vi "2DPlotter.vi"(5 "Reset":bool, 7 "Add":bool, 9 "New Data":i32[][](array[numeric]), 11 "Plot In":i32[][](array[numeric])) -> (3 "Plot Out":i32[][](array[numeric]))   [LabVIEW 2017]
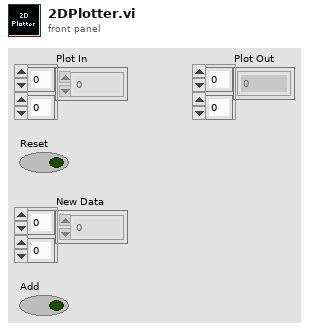
[diagram p1: front panel]
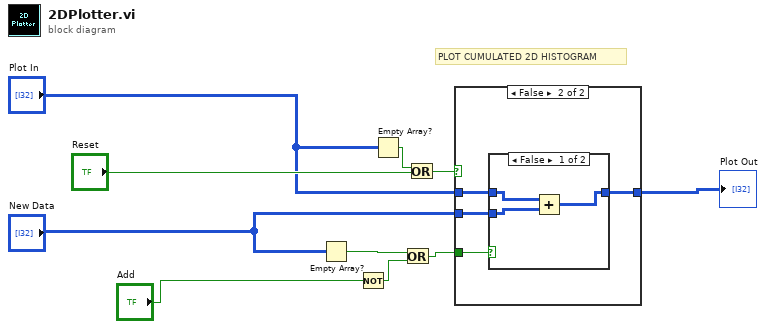
[diagram p0: block diagram]
diagram:
  # "PLOT CUMULATED 2D HISTOGRAM"
  n1 = Empty Array?(array="New Data") -> (empty?=w3:bool)
  n2 = Not(x="Add") -> (.not. x?=w1:bool)
  n3 = Empty Array?(array="Plot In") -> (empty?=w5:bool)
  n4 = Or(x=w3, y=w1) -> (x .or. y?=w2:bool)
  n5 = Or(x=w5, y="Reset") -> (x .or. y?=w4:bool)
  n6 = case shown="False" w4 {
    tunnel: "New Data" -> [w11 w15]
    tunnel: [w11 w14] -> w7
    tunnel: w2 -> [_ w13]
    tunnel: "Plot In" -> [_ w12]
    frame True {
    }
    frame False {
      n7 = case shown="False" w13 {
        tunnel: [w17 w19] -> w14
        tunnel: w15 -> [w18 _]
        tunnel: w12 -> [w16 w19]
        frame False {
          n8 = Add(x=w16, y=w18) -> (x+y=w17:i32[][])
        }
        frame True {
        }
      }
    }
  }
  "Plot Out" <- w7
